vi "enumcase.vi"() -> ()   [LabVIEW 2020]
panel:
  in  "OPERACIONES":T1(ring)
  out "RESULTADO":dbl
  in  "numero 2":dbl
  in  "numero 1":dbl
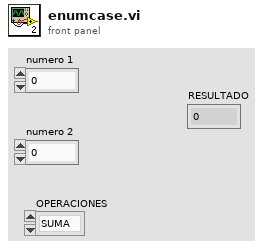
[diagram p1: front panel]
types:
  T1 = enum16{"SUMA", "RESTA", "MULTIPLICACION", "DIVICION"}
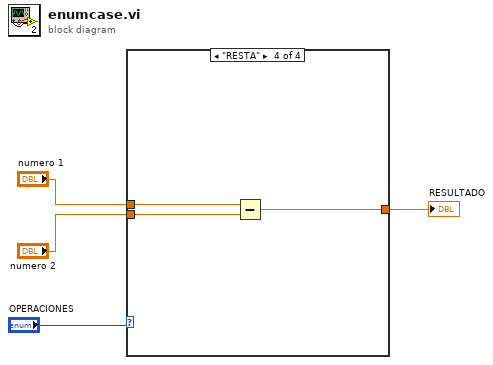
[diagram p0: block diagram]
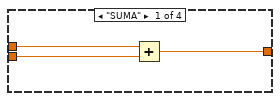
[diagram p2: hidden frame]
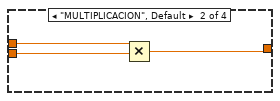
[diagram p3: hidden frame]
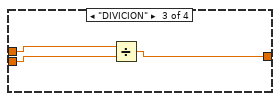
[diagram p4: hidden frame]
diagram:
  n1 = case shown="\"RESTA\"" "OPERACIONES" {
    tunnel: "numero 1" -> [w7 w10 w13 w16]
    tunnel: "numero 2" -> [w6 w9 w12 w15]
    tunnel: [w5 w8 w11 w14] -> w1
    frame "SUMA" {
      n2 = Add(x=w7, y=w6) -> (x+y=w5:dbl)
    }
    frame "MULTIPLICACION", Default {
      n3 = Multiply(x=w10, y=w9) -> (x*y=w8:dbl)
    }
    frame "DIVICION" {
      n4 = Divide(x=w13, y=w12) -> (x/y=w11:dbl)
    }
    frame "RESTA" {
      n5 = Subtract(x=w16, y=w15) -> (x-y=w14:dbl)
    }
  }
  "RESULTADO" <- w1
